vi "AnalogDemultiplex_Multiply.vi"(0 "Analog data cluster":T1) -> (4 "Data A1 out":u64, 6 "Data A2 out":u64)   [LabVIEW 2012]
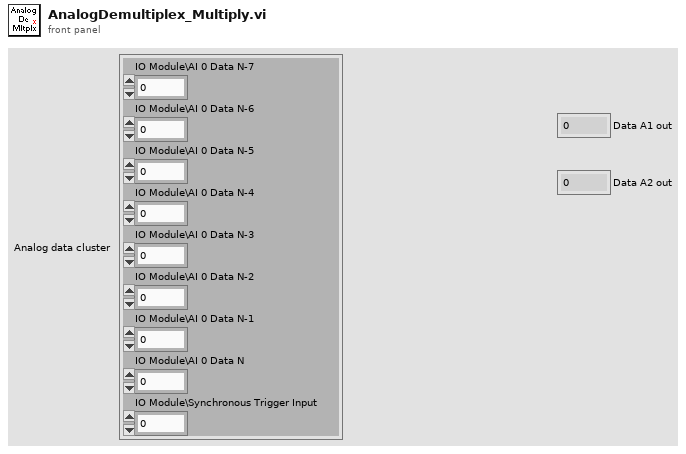
[diagram p1: front panel]
types:
  T1 = cluster{"IO Module\\AI 0 Data N-7":u8, "IO Module\\AI 0 Data N-6":u8, "IO Module\\AI 0 Data N-5":u8, "IO Module\\AI 0 Data N-4":u8, "IO Module\\AI 0 Data N-3":u8, "IO Module\\AI 0 Data N-2":u8, "IO Module\\AI 0 Data N-1":u8, "IO Module\\AI 0 Data N":u8, "IO Module\\Synchronous Trigger Input":u8}
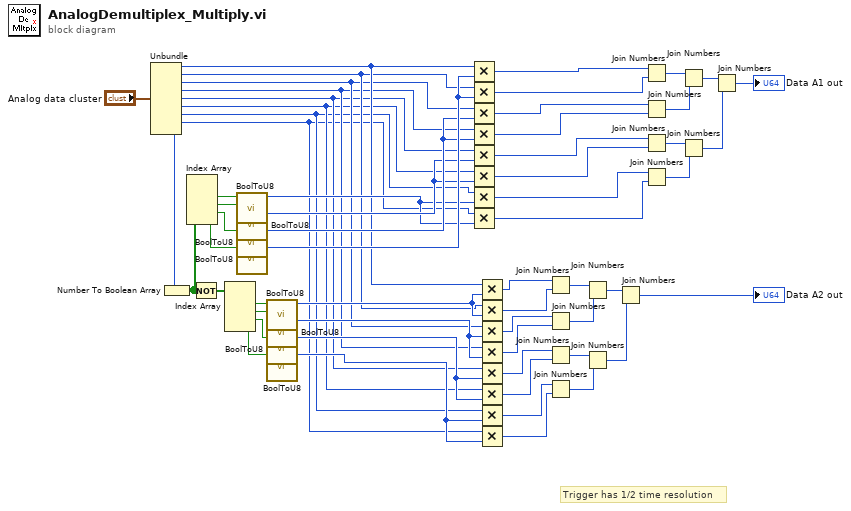
[diagram p0: block diagram]
diagram:
  # "Trigger has 1/2 time resolution"
  n1 = Unbundle("Analog data cluster") -> ("IO Module\\AI 0 Data N-7"=w16:u8, "IO Module\\AI 0 Data N-6"=w15:u8, "IO Module\\AI 0 Data N-5"=w14:u8, "IO Module\\AI 0 Data N-4"=w13:u8, "IO Module\\AI 0 Data N-3"=w12:u8, "IO Module\\AI 0 Data N-2"=w11:u8, "IO Module\\AI 0 Data N-1"=w10:u8, "IO Module\\AI 0 Data N"=w9:u8, "IO Module\\Synchronous Trigger Input"=w42:u8)
  n2 = Number To Boolean Array(number=w42) -> (Boolean array=w33:bool[])
  n3 = Index Array(array=w33) -> (element #1=w37:bool, element #2=w36:bool, element #3=w35:bool, element #4=w34:bool)  [unwired: 4 in]
  n4 = Not(x=w33) -> (.not. x?=w50:bool[])
  n5 = Index Array(array=w50) -> (element #1=w41:bool, element #2=w40:bool, element #3=w39:bool, element #4=w38:bool)  [unwired: 4 in]
  n6 = call "BoolToU8.vi"("Boolean"=w37) -> ("Numeric"=w25:u8)  [unwired: 10 in]
  n7 = call "BoolToU8.vi"("Boolean"=w36) -> ("Numeric"=w26:u8)  [unwired: 10 in]
  n8 = call "BoolToU8.vi"("Boolean"=w35) -> ("Numeric"=w29:u8)  [unwired: 10 in]
  n9 = call "BoolToU8.vi"("Boolean"=w34) -> ("Numeric"=w31:u8)  [unwired: 10 in]
  n10 = call "BoolToU8.vi"("Boolean"=w41) -> ("Numeric"=w20:u8)  [unwired: 10 in]
  n11 = call "BoolToU8.vi"("Boolean"=w40) -> ("Numeric"=w19:u8)  [unwired: 10 in]
  n12 = call "BoolToU8.vi"("Boolean"=w39) -> ("Numeric"=w18:u8)  [unwired: 10 in]
  n13 = call "BoolToU8.vi"("Boolean"=w38) -> ("Numeric"=w17:u8)  [unwired: 10 in]
  n14 = Multiply(x=w16, y=w31) -> (x*y=w32:u8)
  n15 = Multiply(x=w15, y=w31) -> (x*y=w30:u8)
  n16 = Multiply(x=w14, y=w29) -> (x*y=w28:u8)
  n17 = Multiply(x=w13, y=w29) -> (x*y=w27:u8)
  n18 = Multiply(x=w12, y=w26) -> (x*y=w24:u8)
  n19 = Multiply(x=w11, y=w26) -> (x*y=w23:u8)
  n20 = Multiply(x=w10, y=w25) -> (x*y=w21:u8)
  n21 = Multiply(x=w9, y=w25) -> (x*y=w22:u8)
  n22 = Multiply(x=w16, y=w20) -> (x*y=w8:u8)
  n23 = Multiply(x=w15, y=w20) -> (x*y=w7:u8)
  n24 = Multiply(x=w14, y=w19) -> (x*y=w6:u8)
  n25 = Multiply(x=w13, y=w19) -> (x*y=w5:u8)
  n26 = Multiply(x=w12, y=w18) -> (x*y=w3:u8)
  n27 = Multiply(x=w11, y=w18) -> (x*y=w4:u8)
  n28 = Multiply(x=w10, y=w17) -> (x*y=w1:u8)
  n29 = Multiply(x=w9, y=w17) -> (x*y=w2:u8)
  n30 = Join Numbers(hi=w8, lo=w7) -> ((hi.lo)=w51:u16)
  n31 = Join Numbers(hi=w6, lo=w5) -> ((hi.lo)=w52:u16)
  n32 = Join Numbers(hi=w3, lo=w4) -> ((hi.lo)=w53:u16)
  n33 = Join Numbers(hi=w1, lo=w2) -> ((hi.lo)=w54:u16)
  n34 = Join Numbers(hi=w51, lo=w52) -> ((hi.lo)=w56:u32)
  n35 = Join Numbers(hi=w53, lo=w54) -> ((hi.lo)=w55:u32)
  n36 = Join Numbers(hi=w56, lo=w55) -> ((hi.lo)=→"Data A2 out":u64)
  n37 = Join Numbers(hi=w32, lo=w30) -> ((hi.lo)=w44:u16)
  n38 = Join Numbers(hi=w28, lo=w27) -> ((hi.lo)=w45:u16)
  n39 = Join Numbers(hi=w24, lo=w23) -> ((hi.lo)=w46:u16)
  n40 = Join Numbers(hi=w21, lo=w22) -> ((hi.lo)=w47:u16)
  n41 = Join Numbers(hi=w44, lo=w45) -> ((hi.lo)=w49:u32)
  n42 = Join Numbers(hi=w46, lo=w47) -> ((hi.lo)=w48:u32)
  n43 = Join Numbers(hi=w49, lo=w48) -> ((hi.lo)=→"Data A1 out":u64)
